vi "Forward Inbound Message.vi"(8 "error in (no error)":errorcluster, 10 "Inbound Message":refnum<class "PUBLISH.lvclass">, 11 "MQTT Server":refnum<class "Server.lvclass">) -> (0 "error out":errorcluster, 3 "MQTT Server":refnum<class "Server.lvclass">)   [LabVIEW 2013, in "MQTT Server.lvlib" / "Server.lvclass"]
uses:
  Server.lvclass
  <vilib>/LabVIEW Open Source Project/MQTT Control Packets/Control Packets/PUBLISH/PUBLISH.lvclass
  Server.lvclass/Server.ctl
  <vilib>/LabVIEW Open Source Project/MQTT Control Packets/Control Packets/Ack/Ack.lvclass
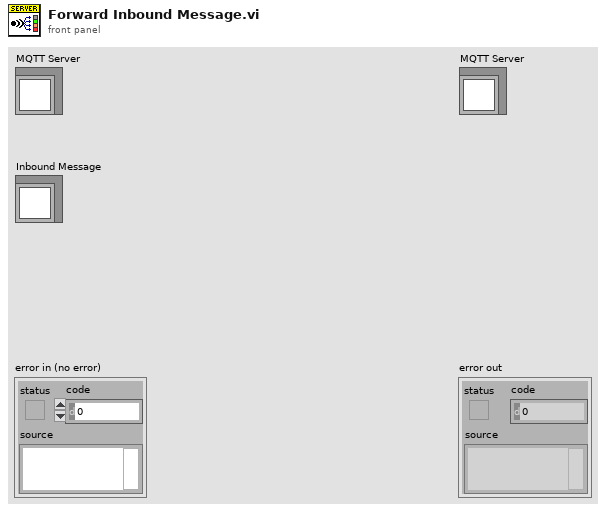
[diagram p1: front panel]
types:
  T1 = typedef "MQTT Server.lvlib/Server.lvclass/Private Events -- cluster.ctl" = cluster{"Inbound Packet":refnum<user-event>, "Inbound Ack":refnum<user-event>}
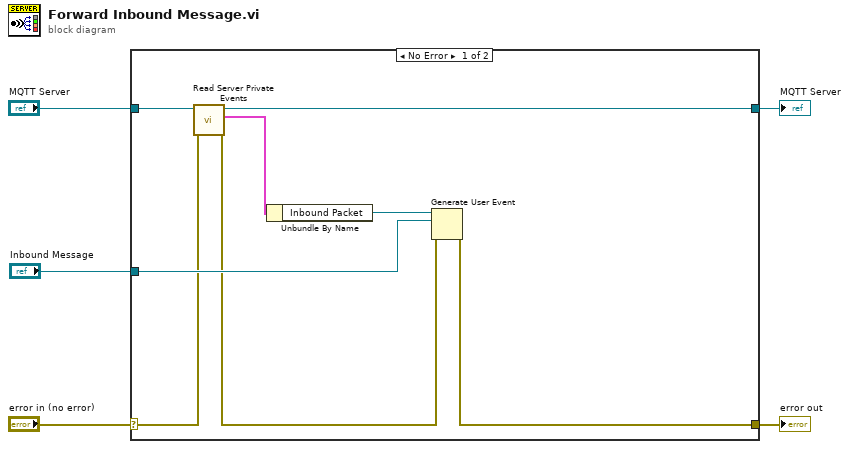
[diagram p0: block diagram]
diagram:
  n1 = case shown="No Error" "error in (no error)" {
    selector: "error in (no error)" -> [w8 w15]
    tunnel: [w13 w15] -> w4
    tunnel: [w9 w14] -> w2
    tunnel: "MQTT Server" -> [w10 w14]
    tunnel: "Inbound Message" -> [w12 _]
    frame No Error {
      n2 = call "Read Server Private Events.vi"("error in (no error)"=w8, "Server in"=w10) -> ("error out"=w7:errorcluster, "Server Private Events"=w6:T1, "Server out"=w9:refnum<class "Server.lvclass">)  [unwired: 7 in]
      n3 = Unbundle By Name(w6) -> ("Inbound Packet"=w11:refnum<user-event>)
      n4 = Generate User Event(user event=w11, event data cluster=w12, error in=w7) -> (error out=w13:errorcluster)  [unwired: 1 in, 1 out]
    }
    frame Error {
    }
  }
  "error out" <- w4
  "MQTT Server" <- w2
